vi "stopAO_img.vi"   [LabVIEW 2015]
uses:
  waveforms/usedAOindepofwf.vi
  Misc/add channel to active arrayv2.vi
  Objects/configuration.vi
  Objects/2pparameters.vi
types:
  T1 = cluster{"AO":refnum<k21>[], "E_AO":errorcluster[]}
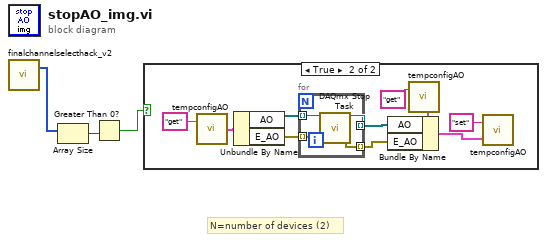
[diagram p0: block diagram]
diagram:
  # "N=number of devices (2)"
  n1 = call "finalchannelselecthack_v2.vi"() -> ("devices"=w1:u32[])  [unwired: 1 in, 1 out]
  n2 = Array Size(array=w1) -> (size(s)=w3:i32)
  n3 = Greater Than 0?(x=w3) -> (x > 0?=w2:bool)
  n4 = case shown="True" w2 {
    frame False {
    }
    frame True {
      n5 = call "tempconfigAO.vi"("command"="get") -> ("Temp Config out"=w12:T1)  [unwired: 1 in]
      n6 = Unbundle By Name(w12) -> ("AO"=w11:refnum<k21>[], "E_AO"=w10:errorcluster[])
      n7 = for {
        tunnel: w11 -> [w17] mode=indexing
        tunnel: w10 -> [w16] mode=indexing
        tunnel: [w15] -> w5 mode=indexing
        tunnel: [w14] -> w4 mode=indexing
        n8 = call <vilib>:"DAQmx Stop Task.vi"("task/channels in"=w17, "error in"=w16) -> ("task out"=w15:refnum<k21>, "error out"=w14:errorcluster)  [unwired: 12 in]
      }
      n9 = call "tempconfigAO.vi"("command"="get") -> ("Temp Config out"=w7:T1)  [unwired: 1 in]
      n10 = Bundle By Name(cluster=w7, "AO"=w5, "E_AO"=w4) -> (w6:T1)
      n11 = call "tempconfigAO.vi"("Temp Config in"=w6, "command"="set") -> ()  [unwired: 1 out]
    }
  }
